vi "AlliGator Decay Fit Output String.vi"(0 "Plot Name":string, 1 "Fit Output":T4={"best nonlinear fit"=[], "best fit parameters"=[], "R^2"=0.0, "RMSE"=0.0, "error out"={"status"=FALSE, "code"=0, "source"=""}, "Fitting Method"=enum."Least Square", "number of function calls"=0, "number of iterations"=0, "covariance"=[], "Chi 2"=0.0, "DOF"=0, "Fit Convergence Criterion"=enum."Continue", "Fitting Algorithm"=enum."Levenberg-Marquardt", "Weighted Fit"=enum."Unweighted", "Gradient"=0.0, "|Delta Chi 2|"=0.0, "|Delta Chi 2|/Chi 2"=0.0, "Max |Delta a| /|a|"=0.0, "Lambda"=-1.0, "RSS"=0.0, "AIC"=0.0, "BIC"=0.0, "Max number of function calls"=0, "Max number of iterations"=0, "IRF"={"X Array"=[], "Y Array"=[]}, "IRF Normalization Factor"=0.0, "Decay Normalization Factor"=0.0, "Number of offset fits"=0, "Weighted Chi2"=-1.0, "Unweighted Chi2"=-1.0}, 2 "All Fit Parameters":dbl[](array[numeric]), 3 "Delta Best Fit Parameters":dbl[](array[numeric]), 4 "Fit Options":T11={"Show Fit Residuals"=TRUE, "Fit Model"=enum."1-Exponential", "Residual Type"=enum."Standard", "Max Decay Percentile"=0.0, "Min Decay Percentile"=0.0, "Show Full Decay"=TRUE, "Weights"=enum."Unweighted", "Fitting Method"=enum."Least Square", "Compute Parameter Uncertainties"=TRUE, "Periodic Boundaries"=TRUE, "Model Calculation"=enum."Simulation", "Period"=1.2500000000000001e-08, "Termination Criteria"={"Max Iterations"=1000, "Max Function Calls"=0, "Max Time"=1000.0, "Function Tolerance"=1e-06, "Parameter Tolerance"=1e-06, "Gradient Tolerance"=0.0, "Min Lambda"=1e-06, "Max Lambda"=1e-06, "Initial Tick Count"=0}, "Offset Resolution"=1.2500000000000001e-08, "Use Local IRF"=TRUE, "Fitting Algorithm"=enum."Levenberg-Marquardt", "Show Confidence Interval "=TRUE, "Confidence Level"=95.0} {"Confidence Level" min=0.0 max=100.0; "Offset Resolution" min=0.0; "Period" min=0.0; "Min Decay Percentile" min=0.0 max=1.0; "Max Decay Percentile" min=0.0 max=100.0}, 5 "Error In":errorcluster, 6 "Plot clipped?":bool, 7 "Guess Parameters":dbl[](array[numeric]), 8 "(Clipped) Plot Range":T3, 9 "Guess Parameters Options":T2=enum."User-provided (normalized)", 10 "Fit Parameter Constraints":T16[](array[typedef]) {"Max Value" format="%#.3g"; "Min Value" format="%#.3g"}, 12 "Decay Plot Interpolation":T1, 13 "CPU (s)":dbl) -> (14 "Fit Output Message":string, 19 "Error Out":errorcluster)   [LabVIEW 2021, in "AlliGator Decay Fit.lvlib"]
doc: "Creates decay fit output string."
uses:
  AlliGator Decay Fit.lvlib
  Fits/IRF(X)PSED/Decay Fit Parameters In List.ctl
  Fits/Fits.lvlib
  <vilib>/ErrorRing/Error Ring.xnode
  <vilib>/Utility/error.llb/DialogType.ctl
  <vilib>/Utility/error.llb/Error Cluster From Error Code.vi
  Fits/IRF(X)PSED/Decay Fit Parameters & Derived Quantities List v2.ctl
  IRF/AlliGator IRF.lvlib
  Fits/Decay Convolution/Decay Model.ctl
  Fits/Residual Type.ctl
  AlliGator Decay Fit Parameter Constraints 2.ctl
  <vilib>/Analysis/Matrix/Datatypes/RealMatrix.ctl
  <vilib>/Analysis/Matrix/NI_Matrix.lvlib
  Fits/Non-linear Fit Output v4.ctl
  Fits/Fit Calculation Method.ctl
  Graphs/Plot Range.ctl
  Graphs/Graphs.lvlib
  Fits/Convergence Criteria.ctl
  Fits/Non-linear Fitting Algorithm.ctl
  AlliGator Guess Parameters Options.ctl
  Fits/Non-linear Fitting Method v2.ctl
  Fits/Nonlinear Fit Method.ctl
  Graphs/XY Graph/XY Graph Plot Data.ctl
  Graphs/XY Graph/XY Graph Add-Ons.lvlib
  Graphs/LabVIEW Plot Interpolation.ctl
  Fits/IRF(X)PSED/Fit Weights Type v2.ctl
  Fits/IRF(X)PSED/Decay Fit Options v4.ctl
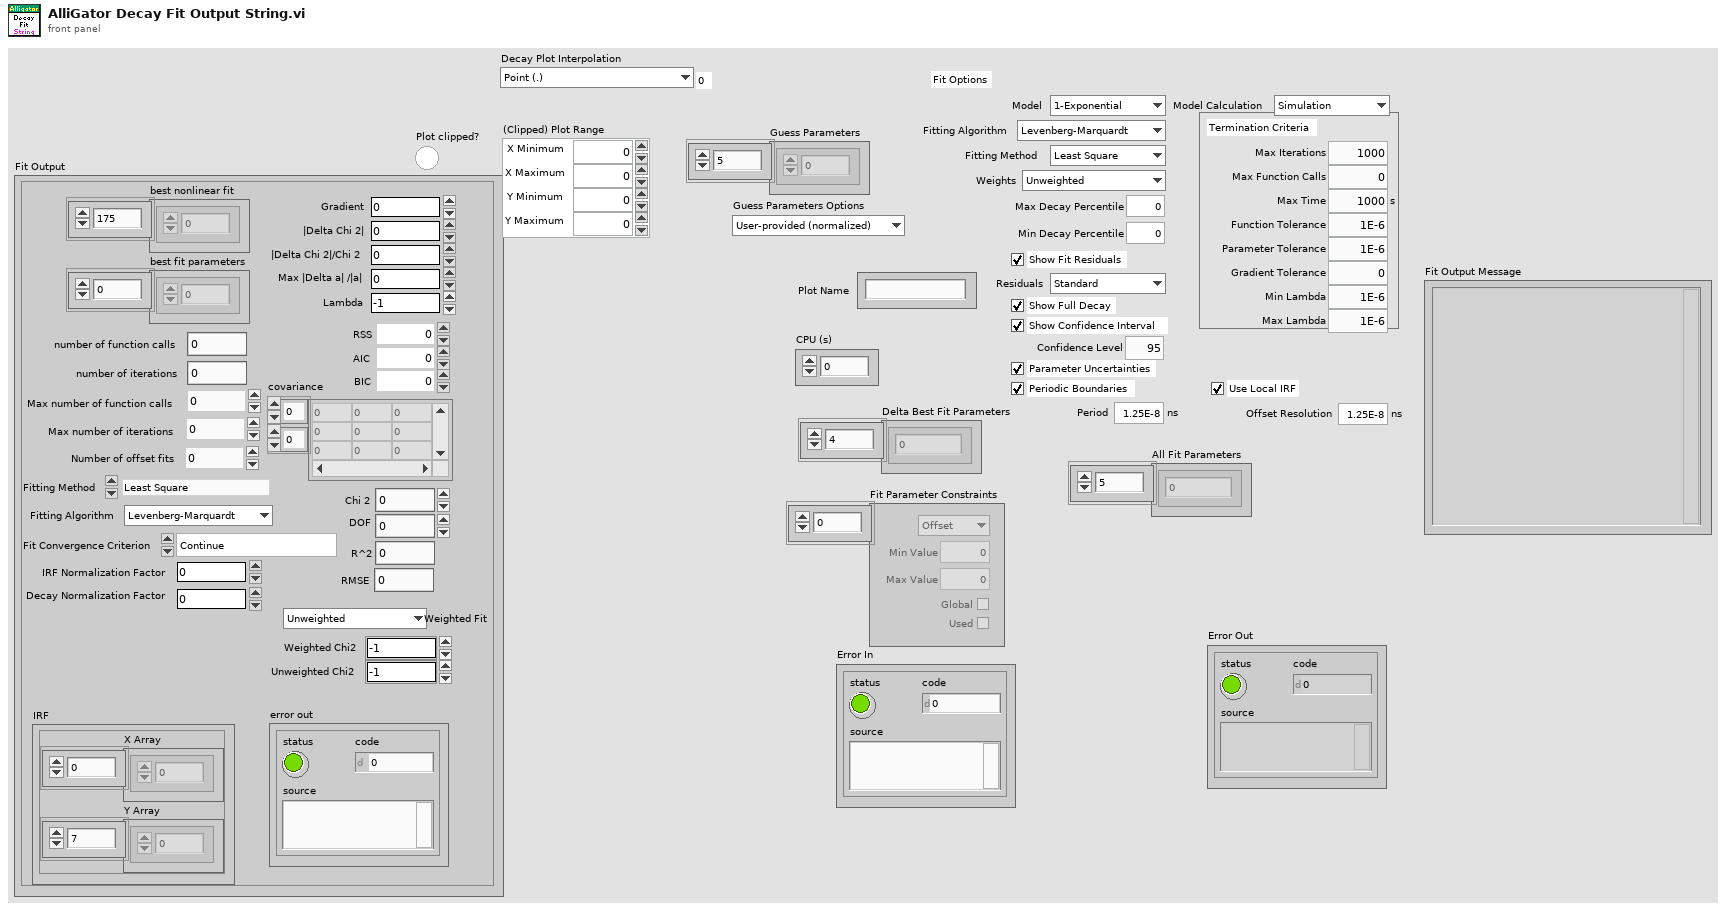
[diagram p1: front panel]
types:
  T1 = typedef "Graphs.lvlib/LabVIEW Plot Interpolation.ctl" = enum16{"Point (.)", "Stepwise Right (--.)", "Line + Point (\\. /)", "Stepwise Left (.--)", "Stepwise Centered (-.-)", "Stepwise Vertical (|.|)", "Line (-)", "Use Previous Plot's Style"}
  T2 = typedef "AlliGator Decay Fit.lvlib/AlliGator Guess Parameters Options.ctl" = enum16{"Numerically estimated", "User-provided", "User-provided (normalized)", "Last valid fitted parameters"}
  T3 = typedef "Graphs.lvlib/Plot Range.ctl" = cluster{"X Minimum":dbl, "X Maximum":dbl, "Y Minimum":dbl, "Y Maximum":dbl}
  T4 = typedef "Fits.lvlib/Non-linear Fit Output v4.ctl" = cluster{"best nonlinear fit":dbl[], "best fit parameters":dbl[], "R^2":dbl, "RMSE":dbl, "error out":errorcluster, "Fitting Method":T5, "number of function calls":i32, "number of iterations":i32, "covariance":T6, "Chi 2":dbl, "DOF":i32, "Fit Convergence Criterion":T7, "Fitting Algorithm":T8, "Weighted Fit":T9, "Gradient":dbl, "|Delta Chi 2|":dbl, "|Delta Chi 2|/Chi 2":dbl, "Max |Delta a| /|a|":dbl, "Lambda":dbl, "RSS":dbl, "AIC":dbl, "BIC":dbl, "Max number of function calls":i32, "Max number of iterations":i32, "IRF":T10, "IRF Normalization Factor":dbl, "Decay Normalization Factor":dbl, "Number of offset fits":i32, "Weighted Chi2":dbl, "Unweighted Chi2":dbl}
  T5 = typedef "Fits.lvlib/Nonlinear Fit Method.ctl" = enum16{"Least Square", "Least Absolute Residual", "Bisquare", "MLE"}
  T6 = typedef "NI_Matrix.lvlib/RealMatrix.ctl" = dbl[][]
  T7 = typedef "Fits.lvlib/Convergence Criteria.ctl" = enum16{"Continue", "Tolerances Exceeded", "Max Time Exceeded", "Max Iterations Exceeded", "Max Function Evaluations Exceeded", "Scale Range Exceeded"}
  T8 = typedef "Fits.lvlib/Non-linear Fitting Algorithm.ctl" = enum16{"Levenberg-Marquardt", "Trust-Region Dogleg"}
  T9 = typedef "Fits.lvlib/Fit Weights Type v2.ctl" = enum16{"Unweighted", "1/Variance (Neyman)", "1/Variance (Pearson)", "Best of All"}
  T10 = typedef "XY Graph Add-Ons.lvlib/XY Graph Plot Data.ctl" = cluster{"X Array":dbl[], "Y Array":dbl[]}
  T11 = typedef "Fits.lvlib/Decay Fit Options v4.ctl" = cluster{"Show Fit Residuals":bool, "Fit Model":T12, "Residual Type":T13, "Max Decay Percentile":dbl, "Min Decay Percentile":dbl, "Show Full Decay":bool, "Weights":T9, "Fitting Method":T14, "Compute Parameter Uncertainties":bool, "Periodic Boundaries":bool, "Model Calculation":T15, "Period":dbl[unit], "Termination Criteria":cluster{"Max Iterations":i32, "Max Function Calls":i32, "Max Time":dbl[unit], "Function Tolerance":dbl, "Parameter Tolerance":dbl, "Gradient Tolerance":dbl, "Min Lambda":dbl, "Max Lambda":dbl, "Initial Tick Count":u32}, "Offset Resolution":dbl[unit], "Use Local IRF":bool, "Fitting Algorithm":T8, "Show Confidence Interval ":bool, "Confidence Level":dbl}
  T12 = typedef "Fits.lvlib/Decay Model.ctl" = enum16{"1-Exponential", "2-Exponentials"}
  T13 = typedef "Fits.lvlib/Residual Type.ctl" = enum16{"Standard", "Normalized", "Reduced"}
  T14 = typedef "Fits.lvlib/Non-linear Fitting Method v2.ctl" = enum16{"Least Square", "Least Absolute Residual", "Bisquare", "MLE", "-", "Best of All"}
  T15 = typedef "Fits.lvlib/Fit Calculation Method.ctl" = enum16{"Simulation", "Convolution", "Integration"}
  T16 = typedef "AlliGator Decay Fit.lvlib/AlliGator Decay Fit Parameter Constraints 2.ctl" = cluster{"Fit Parameter":T17, "Min Value":dbl, "Max Value":dbl, "Global":bool, "Used":bool}
  T17 = typedef "Fits.lvlib/Decay Fit Parameters In List.ctl" = enum16{"Offset", "Baseline", "A_1", "tau_1", "A_2", "tau_2"}
  T18 = cluster{"Max Iterations":i32, "Max Function Calls":i32, "Max Time":dbl[unit], "Function Tolerance":dbl, "Parameter Tolerance":dbl, "Gradient Tolerance":dbl, "Min Lambda":dbl, "Max Lambda":dbl, "Initial Tick Count":u32}
  T19 = typedef "Fits.lvlib/Decay Fit Parameters & Derived Quantities List v2.ctl" = enum16{"Offset", "Baseline", "A_1", "tau_1", "A_2", "tau_2", "<tau>_a", "f1_a", "f2_a", "<tau>_i", "f1_i", "f2_i", "-", "R^2", "Chi^2"}
  T20 = typedef "DialogType.ctl" = u16
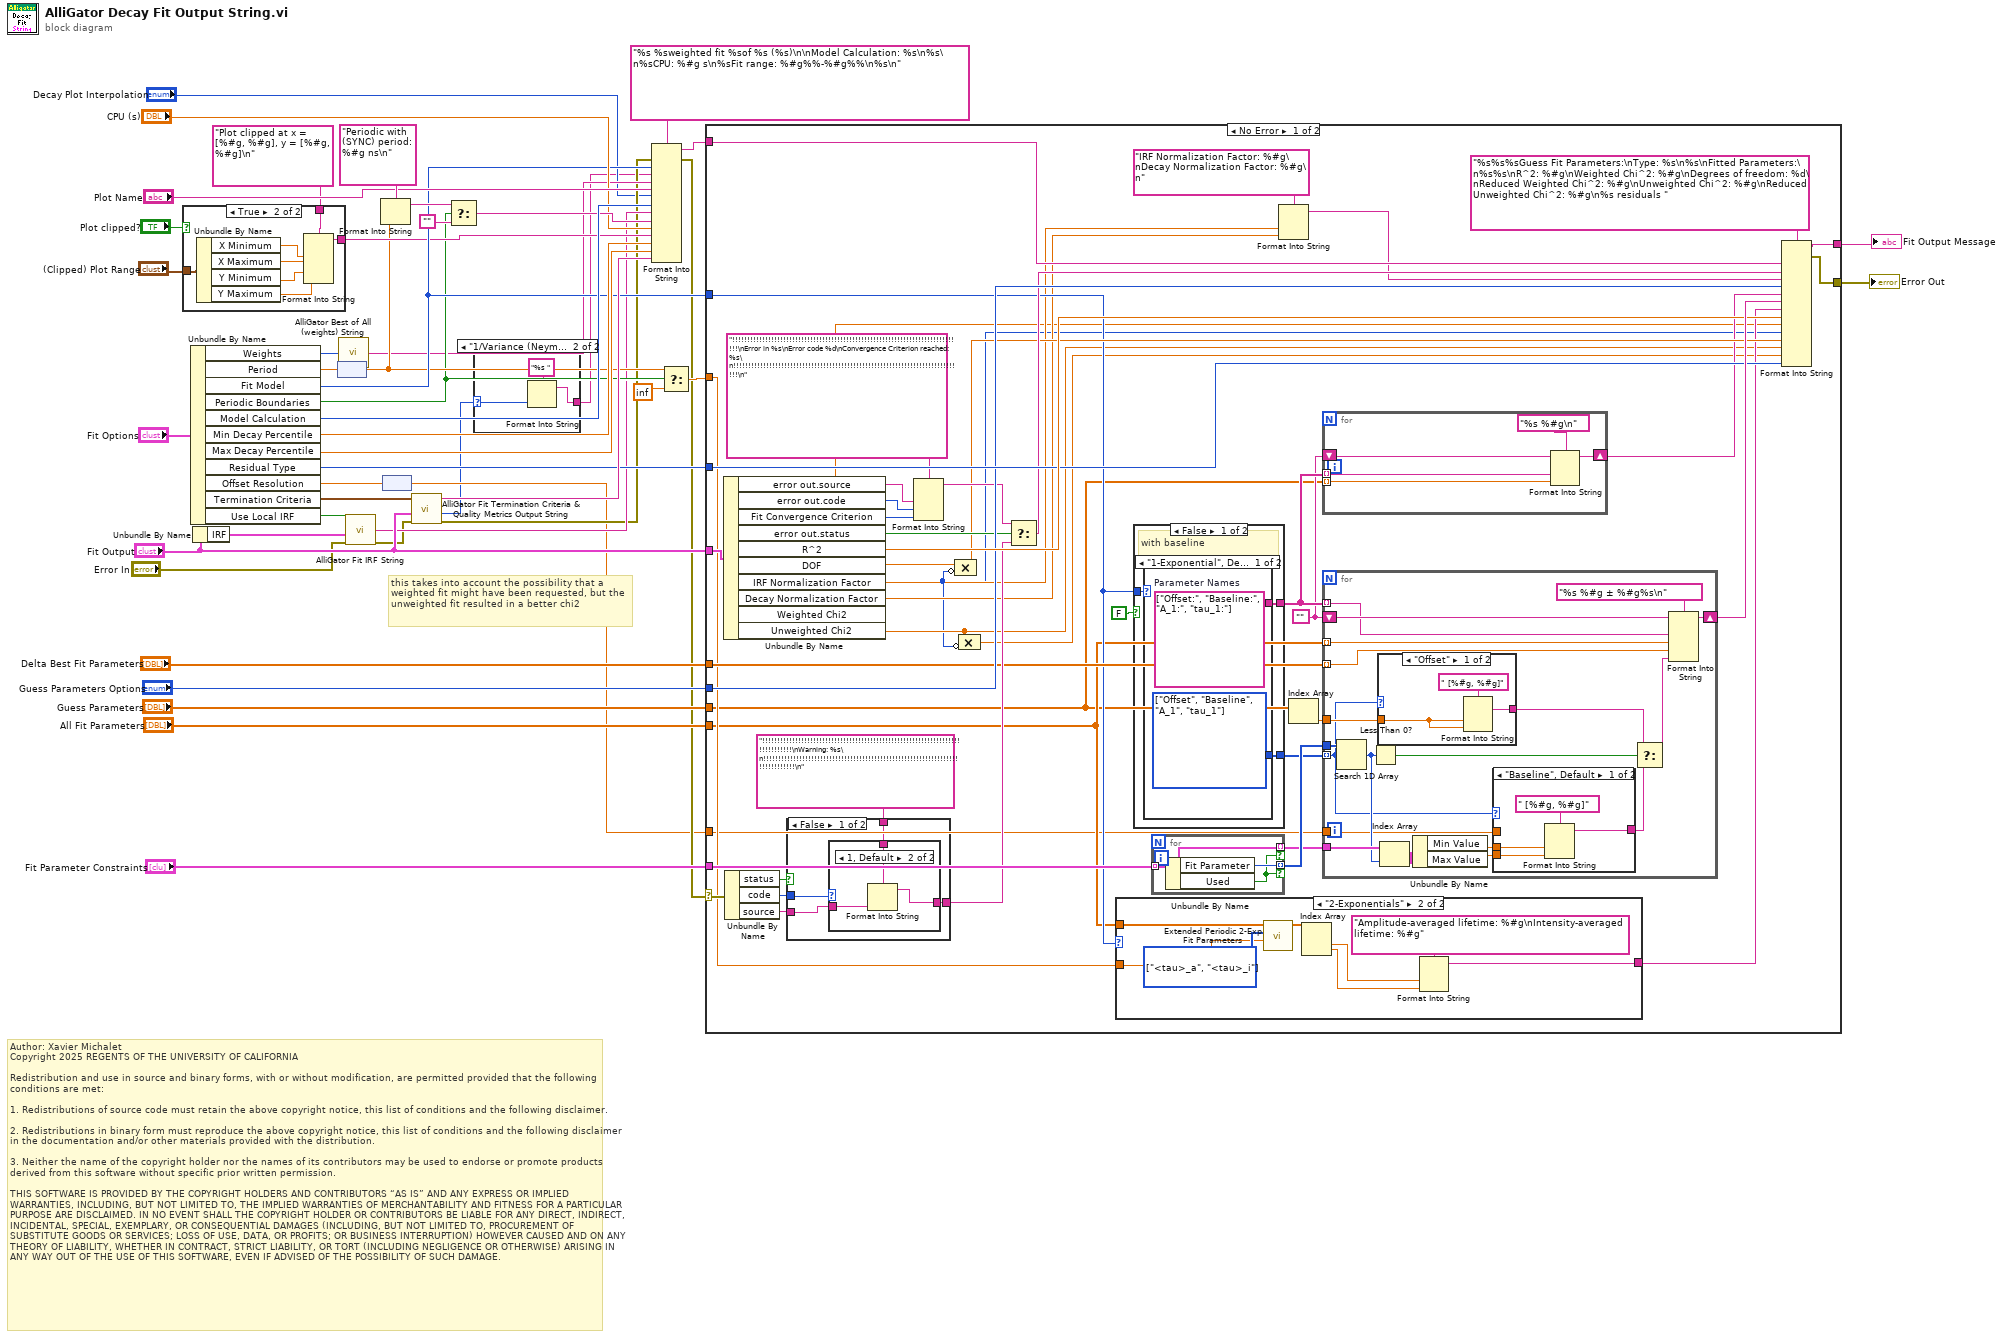
[diagram p0: block diagram]
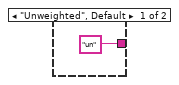
[diagram p2: hidden frame]
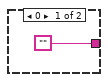
[diagram p5: hidden frame]
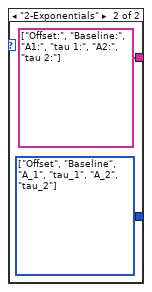
[diagram p7: hidden frame]
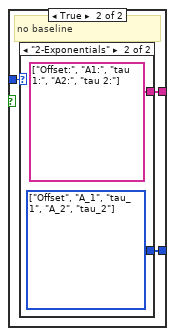
[diagram p8: hidden frame]
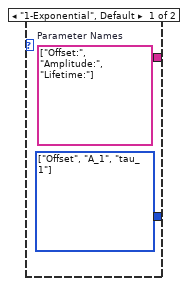
[diagram p9: hidden frame]
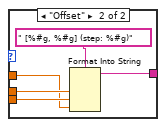
[diagram p10: hidden frame]
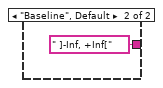
[diagram p11: hidden frame]
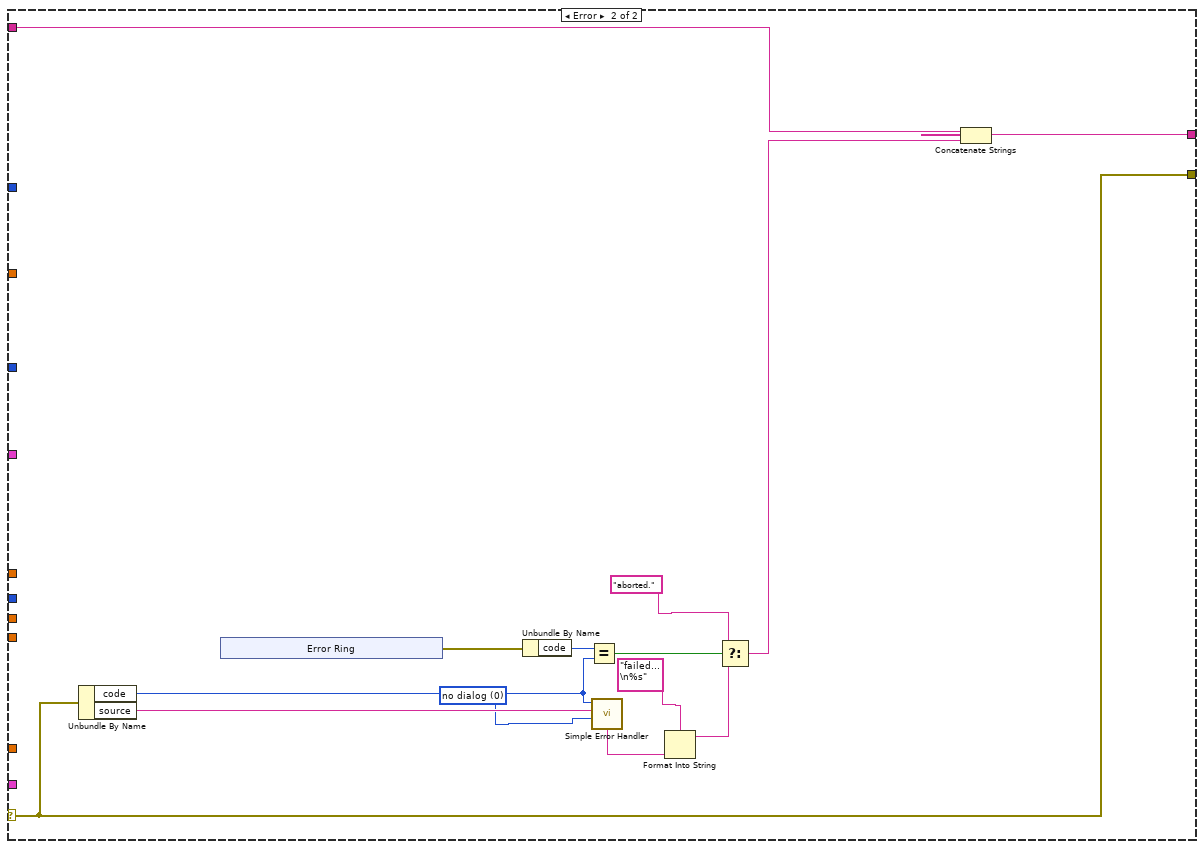
[diagram p12: hidden frame]
diagram:
  # "Author: Xavier Michalet\nCopyright 2025 REGENTS OF THE UNIVERSITY OF CALIFORNIA\n\nRedistribution and use in source and binary forms, with or without modification, are permitted provided that the following conditions are met:\n\n1. Redistributions of source code must retain the above copyright notice, this list of conditions and the following disclaimer.\n\n2. Redistributions in binary form must reproduce the above copyright notice, this list of conditions and the following disclaimer in the documentation and/or other materials provided with the distribution.\n\n3. Neither the name of the copyright holder nor the names of its contributors may be used to endorse or promote products derived from this software without specific prior written permission.\n\nTHIS SOFTWARE IS PROVIDED BY THE COPYRIGHT HOLDERS AND CONTRIBUTORS “AS IS” AND ANY EXPRESS OR IMPLIED WARRANTIES, INCLUDING, BUT NOT LIMITED TO, THE IMPLIED WARRANTIES OF MERCHANTABILITY AND FITNESS FOR A PARTICULAR PURPOSE ARE DISCLAIMED. IN NO EVENT SHALL THE COPYRIGHT HOLDER OR CONTRIBUTORS BE LIABLE FOR ANY DIRECT, INDIRECT, INCIDENTAL, SPECIAL, EXEMPLARY, OR CONSEQUENTIAL DAMAGES (INCLUDING, BUT NOT LIMITED TO, PROCUREMENT OF SUBSTITUTE GOODS OR SERVICES; LOSS OF USE, DATA, OR PROFITS; OR BUSINESS INTERRUPTION) HOWEVER CAUSED AND ON ANY THEORY OF LIABILITY, WHETHER IN CONTRACT, STRICT LIABILITY, OR TORT (INCLUDING NEGLIGENCE OR OTHERWISE) ARISING IN ANY WAY OUT OF THE USE OF THIS SOFTWARE, EVEN IF ADVISED OF THE POSSIBILITY OF SUCH DAMAGE."
  # "this takes into account the possibility that a weighted fit might have been requested, but the unweighted fit resulted in a better chi2"
  n1 = case shown="True" "Plot clipped?" {
    tunnel: "(Clipped) Plot Range" -> [_ w54]
    tunnel: [_ w49] -> w27
    tunnel: "Plot clipped at x = [%#g, %#g], y = [%#g, %#g]\n" ("format string") -> [_ w48]
    frame False {
    }
    frame True {
      n2 = Unbundle By Name(w54) -> ("X Minimum"=w53:dbl, "X Maximum"=w52:dbl, "Y Minimum"=w51:dbl, "Y Maximum"=w50:dbl)
      n3 = Format Into String(format string=w48, w53, w52, w51, w50) -> (resulting string=w49:string)  [unwired: 2 in, 1 out]
    }
  }
  n4 = Unbundle By Name("Fit Options") -> ("Weights"=w16:T9, "Period"=w17:dbl[unit], "Fit Model"=w31:T12, "Periodic Boundaries"=w18:bool, "Model Calculation"=w40:T15, "Min Decay Percentile"=w35:dbl, "Max Decay Percentile"=w34:dbl, "Residual Type"=w30:T13, "Offset Resolution"=w13:dbl[unit], "Termination Criteria"=w14:T18, "Use Local IRF"=w11:bool)
  n5 = Unbundle By Name("Fit Output") -> ("IRF"=w10:T10)
  n6 = node(w17) -> (w23:dbl)
  n7 = call "AlliGator Best of All (weights) String.vi"("Weights"=w16) -> ("Weights String"=w15:string)
  n8 = call "AlliGator Fit IRF String.vi"("Error In"="Error In", "IRF"=w10, "Use Local IRF"=w11) -> ("Error Out"=w8:errorcluster, "IRF String"=w9:string)  [unwired: 7 in]
  n9 = Format Into String(format string="Periodic with (SYNC) period: %#g ns\n", w23) -> (resulting string=w38:string)  [unwired: 2 in, 1 out]
  n10 = node(w13) -> (w4:dbl)
  n11 = call "AlliGator Fit Termination Criteria & Quality Metrics Output String.vi"("Error In"=w8, "Fit Output"="Fit Output", "Termination Criteria"=w14) -> ("Error Out"=w7:errorcluster, "Weighted Fit"=w2:T9, "String"=w33:string)  [unwired: 6 in]
  n12 = Select(t=w38, s=w18, f="") -> (s? t:f=w37:string)
  n13 = case shown="\"1/Variance (Neyman)\"" w2 {
    selector: w2 -> [_ w58]
    tunnel: ["un" w56] -> w1
    frame "Unweighted", Default {
    }
    frame "1/Variance (Neyman)" {
      n14 = Format Into String(format string="%s ", w58) -> (resulting string=w56:string)  [unwired: 2 in, 1 out]
    }
  }
  n15 = Format Into String(format string="%s %sweighted fit %sof %s (%s)\n\nModel Calculation: %s\n%s\n%sCPU: %#g s\n%sFit range: %#g%%-%#g%%\n%s\n", error in=w7, w31, w1, w15, "Plot Name", "Decay Plot Interpolation", w40, w9, w37, "CPU (s)", w27, w35, w34, w33) -> (resulting string=w32:string, error out=w5:errorcluster)  [unwired: 1 in]
  n16 = Select(t=w23, s=w18, f=inf) -> (s? t:f=w21:dbl)
  n17 = case shown="No Error" w5 {
    selector: w5 -> [w99 w176]
    tunnel: "Delta Best Fit Parameters" -> [w77 _]
    tunnel: [w103 w177] -> w46
    tunnel: "Fit Parameter Constraints" -> [w100 _]
    tunnel: "Fit Output" -> [w96 _]
    tunnel: w32 -> [w93 w178]
    tunnel: w31 -> [w73 _]
    tunnel: w30 -> [w92 _]
    tunnel: "Guess Parameters Options" -> [w91 _]
    tunnel: "Guess Parameters" -> [w71 _]
    tunnel: w21 -> [w76 _]
    tunnel: [w74 w176] -> w20
    tunnel: "All Fit Parameters" -> [w72 _]
    tunnel: w4 -> [w67 _]
    frame No Error {
      w79 = ""
      n18 = Unbundle By Name(w96) -> ("error out.source"=w87:string, "error out.code"=w86:i32, "Fit Convergence Criterion"=w82:T7, "error out.status"=w90:bool, "R^2"=w95:dbl, "DOF"=w60:i32, "IRF Normalization Factor"=w64:dbl, "Decay Normalization Factor"=w63:dbl, "Weighted Chi2"=w62:dbl, "Unweighted Chi2"=w61:dbl)
      n19 = Unbundle By Name(w99) -> ("status"=w89:bool, "code"=w98:i32, "source"=w97:string)
      n20 = case shown="False" w89 {
        tunnel: w98 -> [w122 _]
        tunnel: w97 -> [w121 _]
        tunnel: [w120 _] -> w88
        tunnel: "!!!!!!!!!!!!!!!!!!!!!!!!!!!!!!!!!!!!!!!!!!!!!!!!!!!!!!!!!!!!!!!!!!!!!!!!!!!!!\nWarning: %s\n!!!!!!!!!!!!!!!!!!!!!!!!!!!!!!!!!!!!!!!!!!!!!!!!!!!!!!!!!!!!!!!!!!!!!!!!!!!!!\n" ("initial string") -> [w119 _]
        frame False {
          n21 = case shown="1, Default" w122 {
            tunnel: ["" w125] -> w120
            tunnel: w121 -> [_ w126]
            tunnel: w119 -> [_ w124]
            frame 0 {
            }
            frame 1, Default {
              n22 = Format Into String(format string=w124, w126) -> (resulting string=w125:string)  [unwired: 2 in, 1 out]
            }
          }
        }
        frame True {
        }
      }
      n23 = Format Into String(format string="!!!!!!!!!!!!!!!!!!!!!!!!!!!!!!!!!!!!!!!!!!!!!!!!!!!!!!!!!!!!!!!!!!!!!!!!!!!!!\nError in %s\nError code %d\nConvergence Criterion reached: %s\n!!!!!!!!!!!!!!!!!!!!!!!!!!!!!!!!!!!!!!!!!!!!!!!!!!!!!!!!!!!!!!!!!!!!!!!!!!!!!\n", w87, w86, w82) -> (resulting string=w85:string)  [unwired: 2 in, 1 out]
      n24 = Compound Arithmetic op=MULTIPLY(w62, invert w60) -> (w81:dbl)
      n25 = Compound Arithmetic op=MULTIPLY(w61, invert w60) -> (w59:dbl)
      n26 = Select(t=w85, s=w90, f=w88) -> (s? t:f=w84:string)
      n27 = case shown="\"2-Exponentials\"" w73 {
        tunnel: w76 -> [_ w112]
        tunnel: [_ w107] -> w75
        tunnel: w72 -> [_ w106]
        frame "1-Exponential", Default {
        }
        frame "2-Exponentials" {
          w113 = T19[] [enum."<tau>_a", enum."<tau>_i"] items=["Offset", "Baseline", "A_1", "tau_1", "A_2", "tau_2", "<tau>_a", "f1_a", "f2_a", "<tau>_i", "f1_i", "f2_i", "-", "R^2", "Chi^2"] ("Selected Decay Fit Parameter Array")
          n28 = call "Extended Periodic 2-Exp Fit Parameters.vi"("Laser Period"=w112, "Selected Decay Fit Parameter Array"=w113, "Decay Fit Parameters"=w106) -> ("Extended Decay Fit Parameters"=w111:dbl[])  [unwired: 7 in, 1 out]
          n29 = Index Array(array=w111) -> (element #1=w110:dbl, element #2=w109:dbl)  [unwired: 2 in]
          n30 = Format Into String(format string="Amplitude-averaged lifetime: %#g\nIntensity-averaged lifetime: %#g", w110, w109) -> (resulting string=w107:string)  [unwired: 2 in, 1 out]
        }
      }
      n31 = case shown="False" FALSE {
        tunnel: [w129 w136] -> w80
        tunnel: [w128 w135] -> w101
        tunnel: w73 -> [w127 w134]
        frame False {
          # "with baseline"
          n32 = case shown="\"1-Exponential\", Default" w127 {
            tunnel: [w131 string[] ["Offset:", "Baseline:", "A1:", "tau 1:", "A2:", "tau 2:"] ("Parameter Names")] -> w129
            tunnel: [w130 w132] -> w128
            frame "1-Exponential", Default {
              w130 = T17[] [enum."Offset", enum."Baseline", enum."A_1", enum."tau_1"] items=["Offset", "Baseline", "A_1", "tau_1", "A_2", "tau_2"] ("Array")
              w131 = string[] ["Offset:", "Baseline:", "A_1:", "tau_1:"]  # Parameter Names
            }
            frame "2-Exponentials" {
              w132 = T17[] [enum."Offset", enum."Baseline", enum."A_1", enum."tau_1", enum."A_2", enum."tau_2"] items=["Offset", "Baseline", "A_1", "tau_1", "A_2", "tau_2"] ("Array")
            }
          }
        }
        frame True {
          # "no baseline"
          n33 = case shown="\"2-Exponentials\"" w134 {
            tunnel: [w138 string[] ["Offset:", "A1:", "tau 1:", "A2:", "tau 2:"] ("Parameter Names")] -> w136
            tunnel: [w137 w139] -> w135
            frame "1-Exponential", Default {
              w137 = T17[] [enum."Offset", enum."A_1", enum."tau_1"] items=["Offset", "Baseline", "A_1", "tau_1", "A_2", "tau_2"] ("Array")
              w138 = string[] ["Offset:", "Amplitude:", "Lifetime:"]  # Parameter Names
            }
            frame "2-Exponentials" {
              w139 = T17[] [enum."Offset", enum."A_1", enum."tau_1", enum."A_2", enum."tau_2"] items=["Offset", "Baseline", "A_1", "tau_1", "A_2", "tau_2"] ("Array")
            }
          }
        }
      }
      n34 = for {
        tunnel: w100 -> [w142] mode=indexing
        tunnel: [w143] -> w102 mode=indexing if=w141
        tunnel: [w142] -> w69 mode=indexing if=w141
        n35 = Unbundle By Name(w142) -> ("Fit Parameter"=w143:T17, "Used"=w141:bool)
      }
      n36 = Format Into String(format string="IRF Normalization Factor: %#g\nDecay Normalization Factor: %#g\n", w64, w63) -> (resulting string=w65:string)  [unwired: 2 in, 1 out]
      n37 = Index Array(array=w71) -> (element=w70:dbl)  [unwired: 1 in]
      n38 = for {
        tunnel: w80 -> [w118] mode=indexing
        tunnel: w71 -> [w115] mode=indexing
        shift-right: [w114] -> w78
        shift-left: w79 -> [w116]
        n39 = Format Into String(format string="%s %#g\n", initial string=w116, w118, w115) -> (resulting string=w114:string)  [unwired: 1 in, 1 out]
      }
      n40 = for {
        tunnel: w72 -> [w160] mode=indexing
        tunnel: w77 -> [w159] mode=indexing
        tunnel: w80 -> [w148] mode=indexing
        shift-right: [w162] -> w104
        shift-left: w79 -> [w161]
        tunnel: w102 -> [w157]
        tunnel: w101 -> [w145] mode=indexing
        tunnel: w69 -> [w156]
        tunnel: w70 -> [w146]
        tunnel: w67 -> [w144]
        n41 = Search 1D Array(1D array=w157, element=w145) -> (index of element=w149:i32)  [unwired: 1 in]
        n42 = Less Than 0?(x=w149) -> (x < 0?=w155:bool)
        n43 = case shown="\"Offset\"" w145 {
          tunnel: [w174 " ]-Inf, +Inf[" ("format string")] -> w147
          tunnel: w146 -> [w172 _]
          frame "Offset" {
            n44 = Format Into String(format string=" [%#g, %#g]", w172, w172) -> (resulting string=w174:string)  [unwired: 2 in, 1 out]
          }
          frame "Baseline", Default {
          }
        }
        n45 = Index Array(array=w156, index=w149) -> (element=w153:T16)
        n46 = Unbundle By Name(w153) -> ("Min Value"=w152:dbl, "Max Value"=w151:dbl)
        n47 = case shown="\"Baseline\", Default" w145 {
          tunnel: w152 -> [w165 w171]
          tunnel: w151 -> [w164 w170]
          tunnel: [w163 w168] -> w150
          tunnel: w144 -> [_ w167]
          frame "Baseline", Default {
            n48 = Format Into String(format string=" [%#g, %#g]", w165, w164) -> (resulting string=w163:string)  [unwired: 2 in, 1 out]
          }
          frame "Offset" {
            n49 = Format Into String(format string=" [%#g, %#g] (step: %#g)", w171, w170, w167) -> (resulting string=w168:string)  [unwired: 2 in, 1 out]
          }
        }
        n50 = Select(t=w147, s=w155, f=w150) -> (s? t:f=w154:string)
        n51 = Format Into String(format string="%s %#g ± %#g%s\n", initial string=w161, w148, w160, w159, w154) -> (resulting string=w162:string)  [unwired: 1 in, 1 out]
      }
      n52 = Format Into String(format string="%s%s%sGuess Fit Parameters:\nType: %s\n%s\nFitted Parameters:\n%s%s\nR^2: %#g\nWeighted Chi^2: %#g\nDegrees of freedom: %d\nReduced Weighted Chi^2: %#g\nUnweighted Chi^2: %#g\nReduced Unweighted Chi^2: %#g\n%s residuals ", w93, w84, w65, w91, w78, w104, w75, w95, w62, w60, w81, w61, w59, w92) -> (resulting string=w103:string, error out=w74:errorcluster)  [unwired: 2 in]
    }
    frame Error {
      w183 = T20 0 items=["no dialog", "OK message", "continue or stop message", "OK message + warnings", "continue/stop + warnings"] ("type of dialog (OK msg:1)")
      n53 = Unbundle By Name(w176) -> ("code"=w185:i32, "source"=w184:string)
      n54 = xnode "Error Ring"() -> ("error out"=w189:errorcluster)
      n55 = Unbundle By Name(w189) -> ("code"=w188:i32)
      n56 = Equal?(x=w188, y=w185) -> (x = y?=w187:bool)
      n57 = call <vilib>:"Simple Error Handler.vi"("error code (no error:0)"=w185, "error source (\" \")"=w184, "type of dialog (OK msg:1)"=w183) -> ("message"=w181:string)  [unwired: 2 in, 4 out]
      n58 = Format Into String(format string="failed...\n%s", w181) -> (resulting string=w182:string)  [unwired: 2 in, 1 out]
      n59 = Select(t="aborted." ("input 4"), s=w187, f=w182) -> (s? t:f=w179:string)
      n60 = Concatenate Strings(w178, w179) -> (w177:string)
    }
  }
  "Fit Output Message" <- w46
  "Error Out" <- w20
